vi "Create Coverage Report - No Time Stamp - Reports Current Time.vi"() -> ()   [LabVIEW 2017, in "Cobertura.Tests.lvlib"]
uses:
  Cobertura.Tests.lvlib
  Fake Code Coverage/Fake Code Coverage.lvclass
  C:/Users/pasca/Projects/Home/lvunit/CodeCoverage/CodeCoverage.lvclass
  Fake Code Inspector/Fake Code Inspector.lvclass
  C:/Users/pasca/Projects/Home/lvunit/Cobertura/Code Inspector Base/Code Inspector Base.lvclass
  Fake Project Inspector/Fake Project Inspector.lvclass
  C:/Users/pasca/Projects/Home/lvunit/Cobertura/Project Inspector Base/Project Inspector Base.lvclass
  Cobertura/Coverage/Coverage.lvclass/Coverage.ctl
  Cobertura/Coverage/Read Timestamp.vi
  Cobertura/Cobertura.lvlib
  Cobertura/Coverage/Coverage.lvclass
  <vilib>/PNR/Transparent Assertions/Transparent Assertions/Transparent Assertions.lvlib
panel:
  out "error out":errorcluster
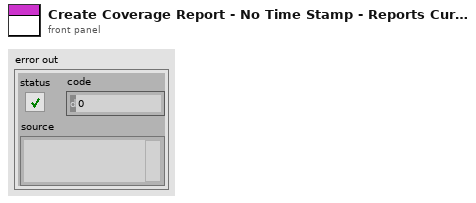
[diagram p1: front panel]
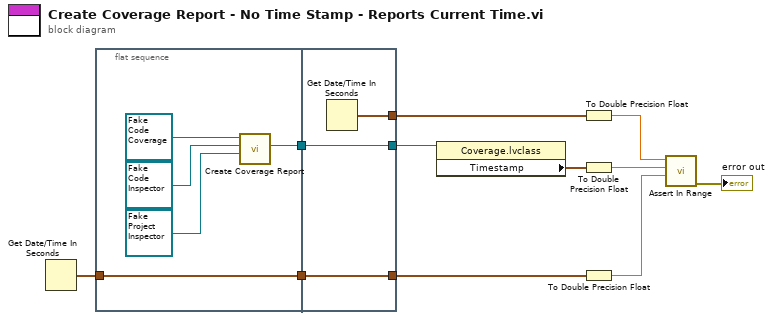
[diagram p0: block diagram]
diagram:
  n1 = Get Date/Time In Seconds() -> (seconds since 1Jan1904=w10:timestamp)
  n2 = flat-sequence {
    tunnel: w10 -> [w12]
    tunnel: [w13] -> w9
    tunnel: [w12] -> w8
    tunnel: [w19] -> w11
    tunnel: w9 -> [w19]
    tunnel: [w18] -> w6
    tunnel: [w17] -> w5
    tunnel: w8 -> [w17]
    frame #0 {
      n3 = call "Create Coverage Report.vi"("Project Inspector"=refnum<class "Fake Project Inspector.lvclass"> refnum ("Cobertura.Tests.lvlib:Fake Project Inspector.lvclass"), "Code Inspector"=refnum<class "Fake Code Inspector.lvclass"> refnum ("Cobertura.Tests.lvlib:Fake Code Inspector.lvclass"), "CodeCoverage in"=refnum<class "Fake Code Coverage.lvclass"> refnum ("Cobertura.Tests.lvlib:Fake Code Coverage.lvclass")) -> ("Coverage"=w13:refnum<class "Coverage.lvclass">)  [unwired: 7 in, 1 out]
    }
    frame #1 {
      n4 = Get Date/Time In Seconds() -> (seconds since 1Jan1904=w18:timestamp)
    }
  }
  n5 = property class="Coverage.lvclass"(reference=w11) -> ("Timestamp"=w7:timestamp)  [unwired: 1 in, 2 out]
  n6 = To Double Precision Float(number=w6) -> (double precision float=w3:dbl)
  n7 = To Double Precision Float(number=w7) -> (double precision float=w4:dbl)
  n8 = To Double Precision Float(number=w5) -> (double precision float=w2:dbl)
  n9 = call <vilib>:"Assert In Range.vi"("Minimum"=w2, "Actual"=w4, "Maximum"=w3) -> ("error out"=→"error out":errorcluster)  [unwired: 8 in]
